vi "7-29-19 Increasing.vi"() -> ()   [LabVIEW 2016]
uses:
  <userlib>/Levylab/LV to ITX/LVtoITX.lvclass
  <vilib>/Analysis/NI_AALPro.lvlib
panel:
  out "dG/dt Vs Temp Normalized":cluster{"Data":dbl[], "Data":dbl[]}[](graph)
  out "Slopes":cluster{dbl[], dbl[]}
  out "G Vs Time Fitted":cluster{"Data":dbl[], "Data":dbl[]}[](graph)
  out "Wavenames":string[](array[string])
  out "G Vs Time":cluster{"Data":dbl[], "Data":dbl[]}[](graph)
  out "Data":dbl[][](array[numeric])
  in  "File Path":path
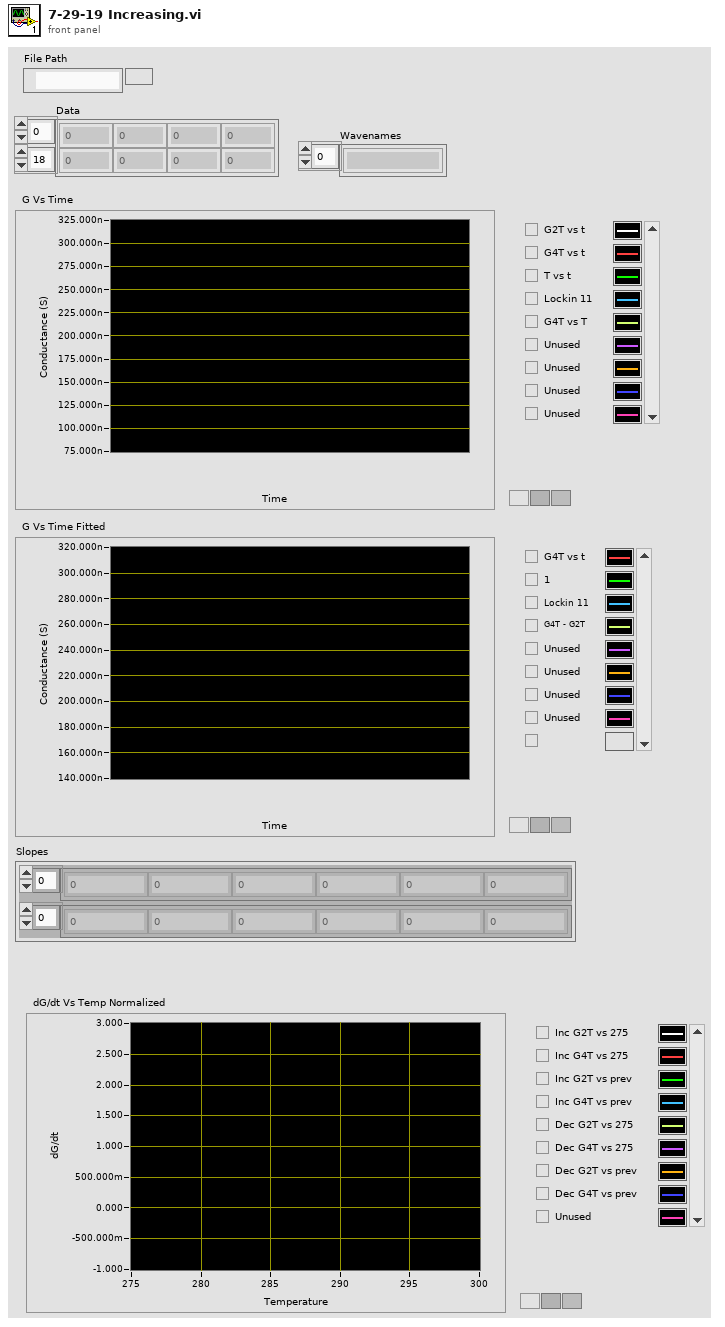
[diagram p1: front panel]
types:
  T1 = cluster{"slope min":dbl, "slope max":dbl, "intercept min":dbl, "intercept max":dbl}
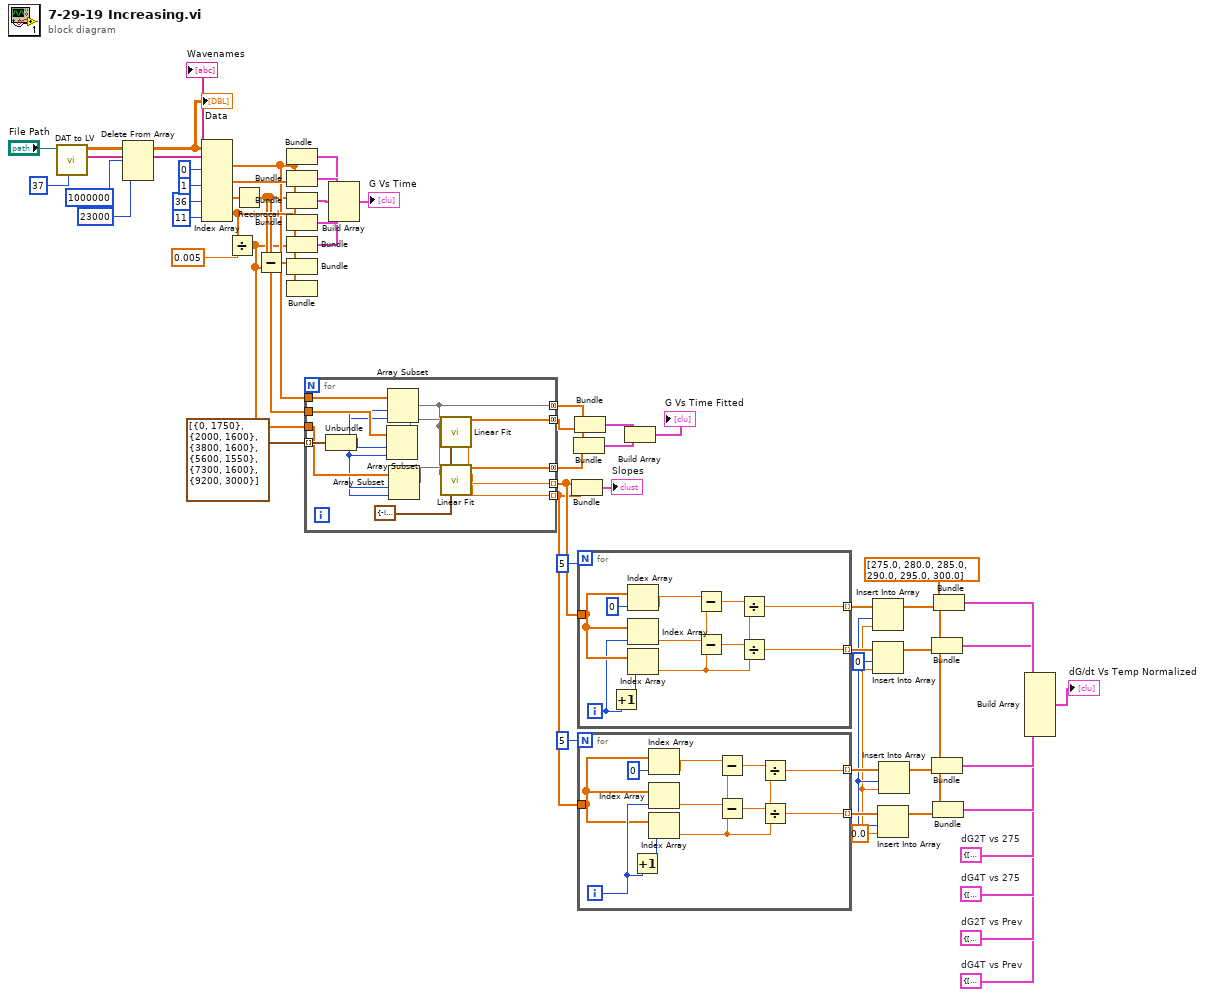
[diagram p0: block diagram]
diagram:
  w2 = cluster{dbl[], dbl[]} {[300.0, 295.0, 290.0, 285.0, 280.0, 275.0], [-0.8359132554427946, -0.6652896480831623, -0.4919979722521102, -0.26330729456953367, -0.0, 0.0]}  # dG2T vs Prev
  w1 = cluster{dbl[], dbl[]} {[300.0, 295.0, 290.0, 285.0, 280.0, 275.0], [2.599254015706807, 1.0398378480849677, 0.5177362302618841, 0.450176702436453, 0.35741808304682104, 0.0]}  # dG4T vs Prev
  w3 = cluster{dbl[], dbl[]} {[300.0, 295.0, 290.0, 285.0, 280.0, 275.0], [2.6352588074829484, 1.0467264910863694, 0.45038429760832155, 0.5167906815284421, 0.3755074501042929, 0.0]}  # dG4T vs 275
  w4 = cluster{dbl[], dbl[]} {[300.0, 295.0, 290.0, 285.0, 280.0, 275.0], [-0.8385386790936263, -0.6695328372151277, -0.5206956162216481, -0.2729955770692637, -0.0, 0.0]}  # dG2T vs 275
  w13 = dbl[] [275.0, 280.0, 285.0, 290.0, 295.0, 300.0]
  w18 = 0.0 ("new element/subarray")
  w19 = 0 ("index")
  n1 = call <userlib>:"DAT to LV.vi"("header length"=37, "File Path"="File Path") -> ("Wavenames"=→"Wavenames":string[], "Data"=w37:dbl[][])  [unwired: 6 in, 2 out]
  n2 = Delete From Array(array=w37, length=1000000, index (row)=23000 ("index")) -> (array with subset deleted=w36:dbl[][])  [unwired: 1 in, 1 out]
  "Data" <- w36
  n3 = Index Array(array=w36, index (col) #1=0 ("disabled index (col)"), index (col) #2=1 ("index (col)"), index (col) #3=36 ("index (col)"), index (col) #4=11 ("index (col)")) -> (element #1=w27:dbl[], element #2=w53:dbl[], element #3=w45:dbl[], element #4=w38:dbl[])  [unwired: 4 in]
  n4 = Divide(x=w38, y=0.005) -> (x/y=w25:dbl[])
  n5 = Reciprocal(x=w45) -> (1/x=w26:dbl[])
  n6 = Subtract(x=w26, y=w25) -> (x-y=w41:dbl[])
  n7 = Bundle("Data"=w27, w25) -> (w44:cluster{"Data":dbl[], dbl[]})  [unwired: 1 in]
  n8 = Bundle("Data"=w27, w26) -> (w52:cluster{"Data":dbl[], dbl[]})  [unwired: 1 in]
  n9 = Bundle("Data"=w27, "Data"=w53) -> (w51:cluster{"Data":dbl[], "Data":dbl[]})  [unwired: 1 in]
  n10 = Bundle("Data"=w27, "Data"=w38) -> (w50:cluster{"Data":dbl[], "Data":dbl[]})  [unwired: 1 in]
  n11 = Bundle("Data"=w27, w41) -> (w42:cluster{"Data":dbl[], dbl[]})  [unwired: 1 in]
  n12 = Bundle("Data"=w53, w25) -> ()  [unwired: 1 in, 1 out]
  n13 = Bundle("Data"=w53, w26) -> ()  [unwired: 1 in, 1 out]
  n14 = for {
    tunnel: cluster{"Index":i32, "Length":i32}[] [{"Index"=0, "Length"=1750}, {"Index"=2000, "Length"=1600}, {"Index"=3800, "Length"=1600}, {"Index"=5600, "Length"=1550}, {"Index"=7300, "Length"=1600}, {"Index"=9200, "Length"=3000}] -> [w71] mode=indexing
    tunnel: w26 -> [w70]
    tunnel: w25 -> [w69]
    tunnel: [w65] -> w32 mode=concatenating
    tunnel: [w64] -> w31 mode=concatenating
    tunnel: [w63] -> w7 mode=indexing
    tunnel: [w62] -> w6 mode=indexing
    tunnel: [w59] -> w33 mode=concatenating
    tunnel: w27 -> [w58]
    w66 = T1 {"slope min"=-inf, "slope max"=inf, "intercept min"=-inf, "intercept max"=inf} ("parameter bounds")
    n15 = Unbundle(w71) -> ("Index"=w68:i32, "Length"=w67:i32)
    n16 = Array Subset(array=w70, index=w68, length=w67) -> (w61:dbl[])
    n17 = Array Subset(array=w58, index=w68, length=w67) -> (w59:dbl[])
    n18 = Array Subset(array=w69, index=w68, length=w67) -> (w60:dbl[])
    n19 = call <vilib>:"Linear Fit.vi"("Y"=w61, "X"=w59, "parameter bounds"=w66) -> ("Best Linear Fit"=w65:dbl[], "slope"=w63:dbl)  [unwired: 8 in, 3 out]
    n20 = call <vilib>:"Linear Fit.vi"("Y"=w60, "X"=w59, "parameter bounds"=w66) -> ("Best Linear Fit"=w64:dbl[], "slope"=w62:dbl)  [unwired: 8 in, 3 out]
  }
  n21 = Build Array(w44, w52, w51, w50, w42) -> (→"G Vs Time":cluster{"Data":dbl[], "Data":dbl[]}[])
  n22 = Bundle(w7, w6) -> (→"Slopes":cluster{dbl[], dbl[]})  [unwired: 1 in]
  n23 = Bundle(w33, "Best Linear Fit"=w31) -> (w30:cluster{dbl[], "Best Linear Fit":dbl[]})  [unwired: 1 in]
  n24 = Bundle(w33, "Best Linear Fit"=w32) -> (w29:cluster{dbl[], "Best Linear Fit":dbl[]})  [unwired: 1 in]
  n25 = for {
    N: 5 -> [_]
    tunnel: w7 -> [w82]
    tunnel: [w73] -> w23 mode=indexing
    tunnel: [w72] -> w22 mode=indexing
    i -> [w80]
    n26 = Increment(x=w80) -> (x+1=w81:i32)
    n27 = Index Array(array=w82, index=0) -> (element=w78:dbl)
    n28 = Index Array(array=w82, index=w80) -> (element=w77:dbl)
    n29 = Index Array(array=w82, index=w81) -> (element=w74:dbl)
    n30 = Subtract(x=w78, y=w74) -> (x-y=w76:dbl)
    n31 = Subtract(x=w77, y=w74) -> (x-y=w75:dbl)
    n32 = Divide(x=w76, y=w74) -> (x/y=w73:dbl)
    n33 = Divide(x=w75, y=w74) -> (x/y=w72:dbl)
  }
  n34 = for {
    N: 5 -> [_]
    tunnel: w6 -> [w85]
    tunnel: [w84] -> w21 mode=indexing
    tunnel: [w83] -> w20 mode=indexing
    i -> [w86]
    n35 = Increment(x=w86) -> (x+1=w87:i32)
    n36 = Index Array(array=w85, index=0) -> (element=w89:dbl)
    n37 = Index Array(array=w85, index=w86) -> (element=w90:dbl)
    n38 = Index Array(array=w85, index=w87) -> (element=w93:dbl)
    n39 = Subtract(x=w89, y=w93) -> (x-y=w91:dbl)
    n40 = Subtract(x=w90, y=w93) -> (x-y=w92:dbl)
    n41 = Divide(x=w91, y=w93) -> (x/y=w84:dbl)
    n42 = Divide(x=w92, y=w93) -> (x/y=w83:dbl)
  }
  n43 = Build Array(w29, w30) -> (→"G Vs Time Fitted":cluster{dbl[], "Best Linear Fit":dbl[]}[])
  n44 = Insert Into Array(array=w23, index=w19, new element=w18) -> (w15:dbl[])
  n45 = Insert Into Array(array=w22, index=w19, new element=w18) -> (w14:dbl[])
  n46 = Insert Into Array(array=w20, index=w19, new element=w18) -> (w16:dbl[])
  n47 = Insert Into Array(array=w21, index=w19, new element=w18) -> (w17:dbl[])
  n48 = Bundle(w13, w14) -> (w10:cluster{dbl[], dbl[]})  [unwired: 1 in]
  n49 = Bundle(w13, w17) -> (w12:cluster{dbl[], dbl[]})  [unwired: 1 in]
  n50 = Bundle(w13, w16) -> (w9:cluster{dbl[], dbl[]})  [unwired: 1 in]
  n51 = Bundle(w13, w15) -> (w11:cluster{dbl[], dbl[]})  [unwired: 1 in]
  n52 = Build Array(w11, w12, w10, w9, w4, w3, w2, w1) -> (→"dG/dt Vs Temp Normalized":cluster{dbl[], dbl[]}[])
